vi "PH_Cont-601k_PSU.set Hard- and Software to GUI.vi"(0 "VI in":refnum<vi>, 2 "Hard- and Software":T1={"VISA resource"="COM1", "Driver Revision"="", "Firmware Revision"=""}, 3 "Blinking? (False)":bool, 5 "error in (no error)":errorcluster) -> (14 "VI out":refnum<vi>, 19 "error out":errorcluster)   [LabVIEW 2014, in "PH_Cont-601k_PSU.lvlib"]
uses:
  PH_Cont-601k_PSU.lvlib
  PH_Cont-601k_PSU.Device Informaton.ctl
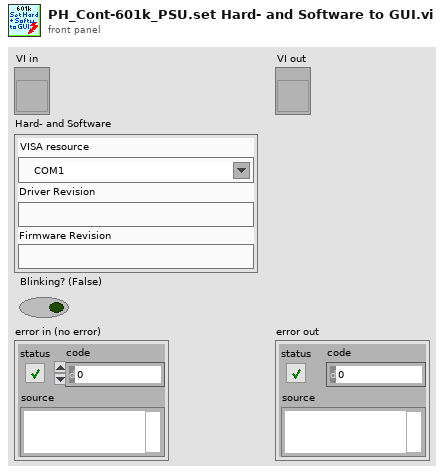
[diagram p1: front panel]
types:
  T1 = typedef "PH_Cont-601k_PSU.lvlib/PH_Cont-601k_PSU.Device Informaton.ctl" = cluster{"VISA resource":refnum<visa-resource-name>, "Driver Revision":string, "Firmware Revision":string}
  T2 = typedef "PH_Cont-601k_PSU.lvlib/PH_Cont-601k_PSU.i attribute.ctl" = cluster{"GUI Refs":T3, "Interlock":bool, "Service ID applied Voltage":i32, "Device Settings":cluster{"Configuration":T4, "Flash Interval [s]":dbl, "Mode":T5, "Voltage [V]":u16, "Charge":bool, "VISA resource name":refnum<visa-resource-name>}, "Readyness":T6, "Information":cluster{"VISA resource name":refnum<visa-resource-name>, "Tagname Power On":string, "Interlock":cluster{"Instance":string, "Tagname":string}, "Limits [V]":cluster{"Lower":dbl, "Upper":dbl}, "Tagname PSU On":string}, "R2S":bool, "Charge is allowed":bool}
  T3 = typedef "PH_Cont-601k_PSU.lvlib/PH_Cont-601k_PSU.GUI Refs.ctl" = cluster{"Power On":refnum<vi>, "Hard- and Software":refnum<vi>, "Device Status":refnum<vi>, "Device Error":refnum<vi>, "Configuration":refnum<vi>, "Flash Interval [s]":refnum<vi>, "Interlock":refnum<vi>, "Interlock Indicator":refnum<vi>, "Voltage [V]":refnum<vi>, "Readyness":refnum<vi>, "Mode":refnum<vi>, "Reset Error":refnum<vi>, "Expert working":refnum<vi>, "Charge":refnum<vi>, "PSU On":refnum<vi>}
  T4 = typedef "PH_Cont-601k_PSU.lvlib/PH_Cont-601k_PSU.Configuration.ctl" = u16
  T5 = typedef "PH_Cont-601k_PSU.lvlib/PH_Cont-601k_PSU.Mode.ctl" = enum32{"STOP", "STANDBY", "READY", "EMISSION", "ERROR"}
  T6 = typedef "PH_Cont-601k_PSU.lvlib/PH_Cont-601k_PSU.Readyness.ctl" = cluster{"Program":T7, "Device":T8}
  T7 = typedef "PH_Cont-601k_PSU.lvlib/PH_Cont-601k_PSU.Readyness Program.ctl" = enum32{"OFF", "POWER", "INTERLOCK"}
  T8 = typedef "PH_Cont-601k_PSU.lvlib/PH_Cont-601k_PSU.Readyness Device.ctl" = enum32{"OFF", "CONNECTING", "CONNECTED", "OPERATING", "EOC", "ERROR"}
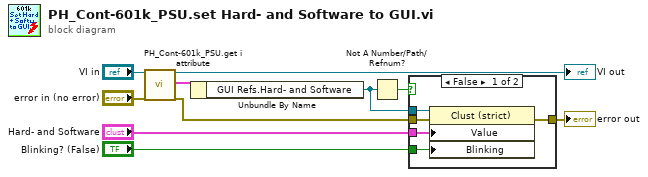
[diagram p0: block diagram]
diagram:
  n1 = call "PH_Cont-601k_PSU.get i attribute.vi"("i ref in"="VI in", "error in (no error)"="error in (no error)") -> ("i ref out"=→"VI out":refnum<vi>, "i attribute"=w6:T2, "error out"=w8:errorcluster)  [unwired: 15 in]
  n2 = Unbundle By Name(w6) -> ("GUI Refs.Hard- and Software"=w3:refnum<vi>)
  n3 = Not A Number/Path/Refnum?(number/path/refnum=w3) -> (NaN/Path/Refnum?=w4:bool)
  n4 = case shown="False" w4 {
    tunnel: w8 -> [w15 w16]
    tunnel: [w14 w16] -> w5
    tunnel: w3 -> [w13 _]
    tunnel: "Hard- and Software" -> [w12 _]
    tunnel: "Blinking? (False)" -> [w11 _]
    frame False {
      n5 = property class="Clust (strict)"(reference=w13, error in=w15, "Value"=w12, "Blinking"=w11) -> (error out=w14:errorcluster)  [unwired: 1 out]
    }
    frame True {
    }
  }
  "error out" <- w5
